vi "GetText.vi"(8 "error in":errorcluster, 11 "voltage in":refnum<class "Voltage.lvclass">) -> (0 "error out":errorcluster, 1 "additional text":string, 2 "text":string, 3 "voltage out":refnum<class "Voltage.lvclass">, 4 "glyph":string)   [LabVIEW 2015, in "Voltage.lvclass"]
uses:
  Voltage.lvclass
  Channel/Channel.lvclass
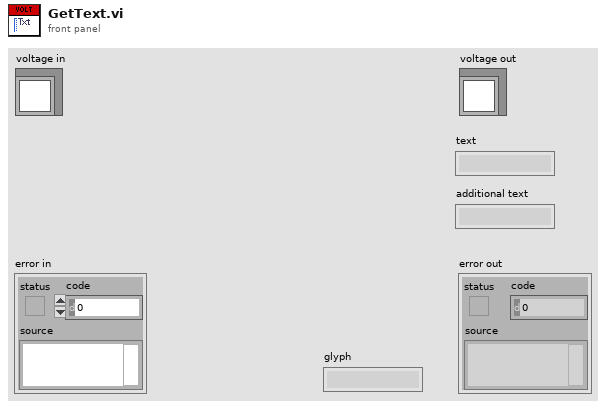
[diagram p1: front panel]
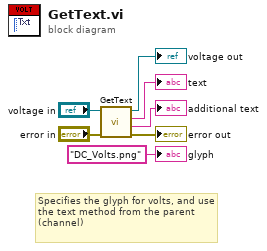
[diagram p0: block diagram]
diagram:
  # "Specifies the glyph for volts, and use the text method from the parent (channel)"
  n1 = call-parent "GetText.vi"("error in"="error in", "channel in"="voltage in") -> ("error out"=→"error out":errorcluster, "additional text"=→"additional text":string, "text"=→"text":string, "channel out"=→"voltage out":refnum<class "Voltage.lvclass">)  [unwired: 5 in, 1 out]
  "glyph" <- "DC_Volts.png" ("glyph")
